vi "MAG3110 Test Program.vi"() -> ()   [LabVIEW 2012]
panel:
  out "Z (uT)":dbl
  out "Y (uT)":dbl
  out "X (uT)":dbl
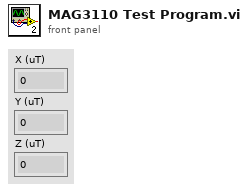
[diagram p1: front panel]
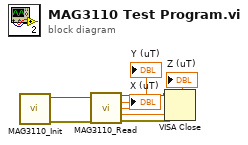
[diagram p0: block diagram]
diagram:
  n1 = call "MAG3110_Init.vi"() -> ("VISA resource name out"=w7:refnum<visa-resource-name>, "error out"=w5:errorcluster)  [unwired: 9 in]
  n2 = call "MAG3110_Read.vi"("VISA resource name"=w7, "error in (no error)"=w5) -> ("VISA resource name out"=w6:refnum<visa-resource-name>, "X (uT)"=→"X (uT)":dbl, "Y (uT)"=→"Y (uT)":dbl, "Z (uT)"=→"Z (uT)":dbl, "error out"=w4:errorcluster)  [unwired: 9 in]
  n3 = VISA Close(VISA resource name=w6, error in (no error)=w4) -> ()  [unwired: 1 out]
